vi "Main.vi"(1 "Wait (ms)":dbl, 2 "Input Expression":string) -> (0 "Evaluation":string[](array[string]))   [LabVIEW 2012]
uses:
  <vilib>/regexp/Match Regular Expression.xnode
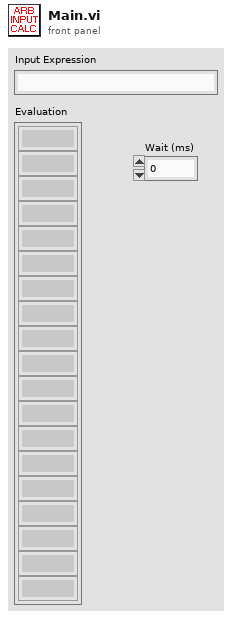
[diagram p1: front panel]
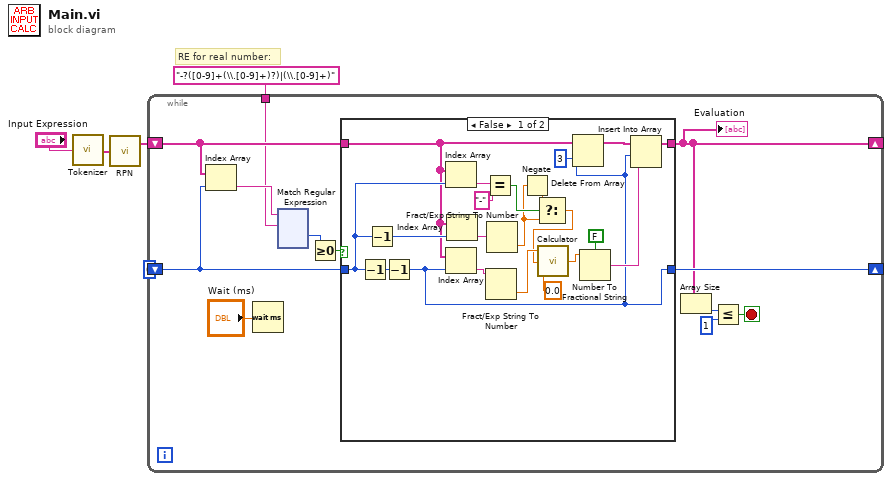
[diagram p0: block diagram]
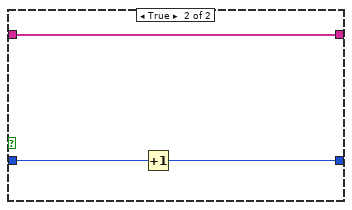
[diagram p2: hidden frame]
diagram:
  # "RE for real number:"
  n1 = call "Tokenizer.vi"("Input String"="Input Expression") -> ("Tokenized Array"=w4:string[])
  n2 = call "RPN.vi"("Input stack\n(tokenized)"=w4) -> ("Output Queue"=w2:string[])  [unwired: 1 out]
  n3 = while {
    shift-right: [w8] -> _
    shift-left: w2 -> [w10]
    shift-right: [w16] -> _
    shift-left: 0 ("index") -> [w9]
    tunnel: "-?([0-9]+(\\.[0-9]+)?)|(\\.[0-9]+)" -> [w7]
    stop <- w11 stop-if-true
    n4 = Index Array(array=w10, index=w9) -> (element=w17:string)
    n5 = Wait (ms)(milliseconds to wait="Wait (ms)") -> ()  [unwired: 1 out]
    n6 = xnode "Match Regular Expression"("input string"=w17, "regular expression"=w7) -> ("offset past match"=w15:i32)  [unwired: 4 in, 4 out]
    n7 = Greater Or Equal To 0?(x=w15) -> (x >= 0?=w14:bool)
    n8 = case shown="False" w14 {
      tunnel: w9 -> [w35 w41]
      tunnel: [w30 w40] -> w16
      tunnel: w10 -> [w34 w39]
      tunnel: [w32 w39] -> w8
      frame False {
        n9 = Decrement(x=w35) -> (x-1=w38:i32)
        n10 = Decrement(x=w35) -> (x-1=w36:i32)
        n11 = Decrement(x=w38) -> (x-1=w30:i32)
        n12 = Index Array(array=w34, index=w35) -> (element=w26:string)
        n13 = Index Array(array=w34, index=w30) -> (element=w27:string)
        n14 = Index Array(array=w34, index=w36) -> (element=w28:string)
        n15 = Equal?(x=w26, y="-") -> (x = y?=w24:bool)
        n16 = Fract/Exp String To Number(string=w27) -> (number=w21:dbl)  [unwired: 3 in, 1 out]
        n17 = Fract/Exp String To Number(string=w28) -> (number=w23:dbl)  [unwired: 3 in, 1 out]
        n18 = Negate(x=w23) -> (-x=w22:dbl)
        n19 = Select(t=w22, s=w24, f=w23) -> (s? t:f=w20:dbl)
        n20 = call "Calculator.vi"("Wait (ms)"=0.0, "Input 2"=w20, "Input 1"=w21) -> ("Decimal Result"=w18:dbl)
        n21 = Delete From Array(array=w34, length=3, index=w30) -> (array with subset deleted=w33:string[])  [unwired: 1 out]
        n22 = Number To Fractional String(use system decimal point (T)=FALSE, number=w18) -> (F-format string=w31:string)  [unwired: 2 in]
        n23 = Insert Into Array(array=w33, index=w30, new element=w31) -> (w32:string[])
      }
      frame True {
        n24 = Increment(x=w41) -> (x+1=w40:i32)
      }
    }
    "Evaluation" <- w8
    n25 = Array Size(array=w8) -> (size(s)=w13:i32)
    n26 = Less Or Equal?(x=w13, y=1) -> (x <= y?=w11:bool)
  }
